vi "FisherPaykel Check SubCycle.vi"(7 "Agitate Parameters Settle Stroke":T1={"Agitate Running Time (sec)"=15, "Direction (CW or CCW)"="1", "RampUpTime (1-600ms)"=250, "TargetSpeed (0-200RPM)"=726, "PlateauTime (0-1800ms 10ms Increment)"=1000, "PauseTime (0-1800ms 10ms Increment)"=600} {"PauseTime (0-1800ms 10ms Increment)" step=10; "PlateauTime (0-1800ms 10ms Increment)" step=10; "TargetSpeed (0-200RPM)" max=1600 step=1; "RampUpTime (1-600ms)" max=600 step=10; "Agitate Running Time (sec)" step=1}, 8 "Error In":errorcluster, 9 "Agitate Parameters":T1={"Agitate Running Time (sec)"=0, "Direction (CW or CCW)"="0", "RampUpTime (1-600ms)"=0, "TargetSpeed (0-200RPM)"=0, "PlateauTime (0-1800ms 10ms Increment)"=0, "PauseTime (0-1800ms 10ms Increment)"=0} {"PauseTime (0-1800ms 10ms Increment)" step=10; "PlateauTime (0-1800ms 10ms Increment)" step=10; "TargetSpeed (0-200RPM)" max=1600 step=1; "RampUpTime (1-600ms)" max=600 step=10; "Agitate Running Time (sec)" step=1}, 10 "Spin Profile":T3={"Target Speed (RPM)"=23, "Acceleration Rate - (10 Slowest/1000 Fastest)"=10, "Running Time (s)"=20, "Direction (CW or CCW)"=""} {"Running Time (s)" step=1; "Acceleration Rate - (10 Slowest/1000 Fastest)" min=10 max=1000 step=1; "Target Speed (RPM)" min=23 max=1600 step=1}, 11 "ERD Array":string[][](array[string])=[["Motor Profile Status (0xF0B7)", "Started"], ["Motor Profile (0xF0B7)", "9"], ["Motor Mode (0xF0B1)", "Idle"], ["Mode Shift Status (0xFF22)", "Agitate State"], ["Sub-Cycle (0xF07B)", "WASH"], ["Remaining Cycle Time(s) (0xF061)", "1707"], ["Target Speed (RPM) (0xF0AC)", "0"]]) -> (0 "Error Out":errorcluster, 1 "Agitate Parameters Output":T1={"Agitate Running Time (sec)"=0, "Direction (CW or CCW)"="0", "RampUpTime (1-600ms)"=0, "TargetSpeed (0-200RPM)"=0, "PlateauTime (0-1800ms 10ms Increment)"=0, "PauseTime (0-1800ms 10ms Increment)"=0} {"PauseTime (0-1800ms 10ms Increment)" step=10; "PlateauTime (0-1800ms 10ms Increment)" step=10; "TargetSpeed (0-200RPM)" max=1600 step=1; "RampUpTime (1-600ms)" max=600 step=10; "Agitate Running Time (sec)" step=1}, 2 "Spin Profile Output":T3={"Target Speed (RPM)"=23, "Acceleration Rate - (10 Slowest/1000 Fastest)"=10, "Running Time (s)"=20, "Direction (CW or CCW)"=""} {"Running Time (s)" step=1; "Acceleration Rate - (10 Slowest/1000 Fastest)" min=10 max=1000 step=1; "Target Speed (RPM)" min=23 max=1600 step=1}, 3 "States Output":string)   [LabVIEW 2016]
uses:
  Type Definitions/Fisher Paykel Motor Profile.ctl
  Type Definitions/FisherPaykel Direction CMD.ctl
  Type Definitions/Fisher Paykel Agitate Parameters.ctl
panel:
  # "Agitate Profile Parameters"
  # "Agitate Start Parameters"
  # "Agitate Profile Parameters"
  # "Agitate Start Parameters"
  # "Agitate Profile Parameters"
  # "Agitate Start Parameters"
  # "Spin Profile Parameters"
  # "Spin Start Parameters"
  # "Spin Profile Parameters"
  # "Spin Start Parameters"
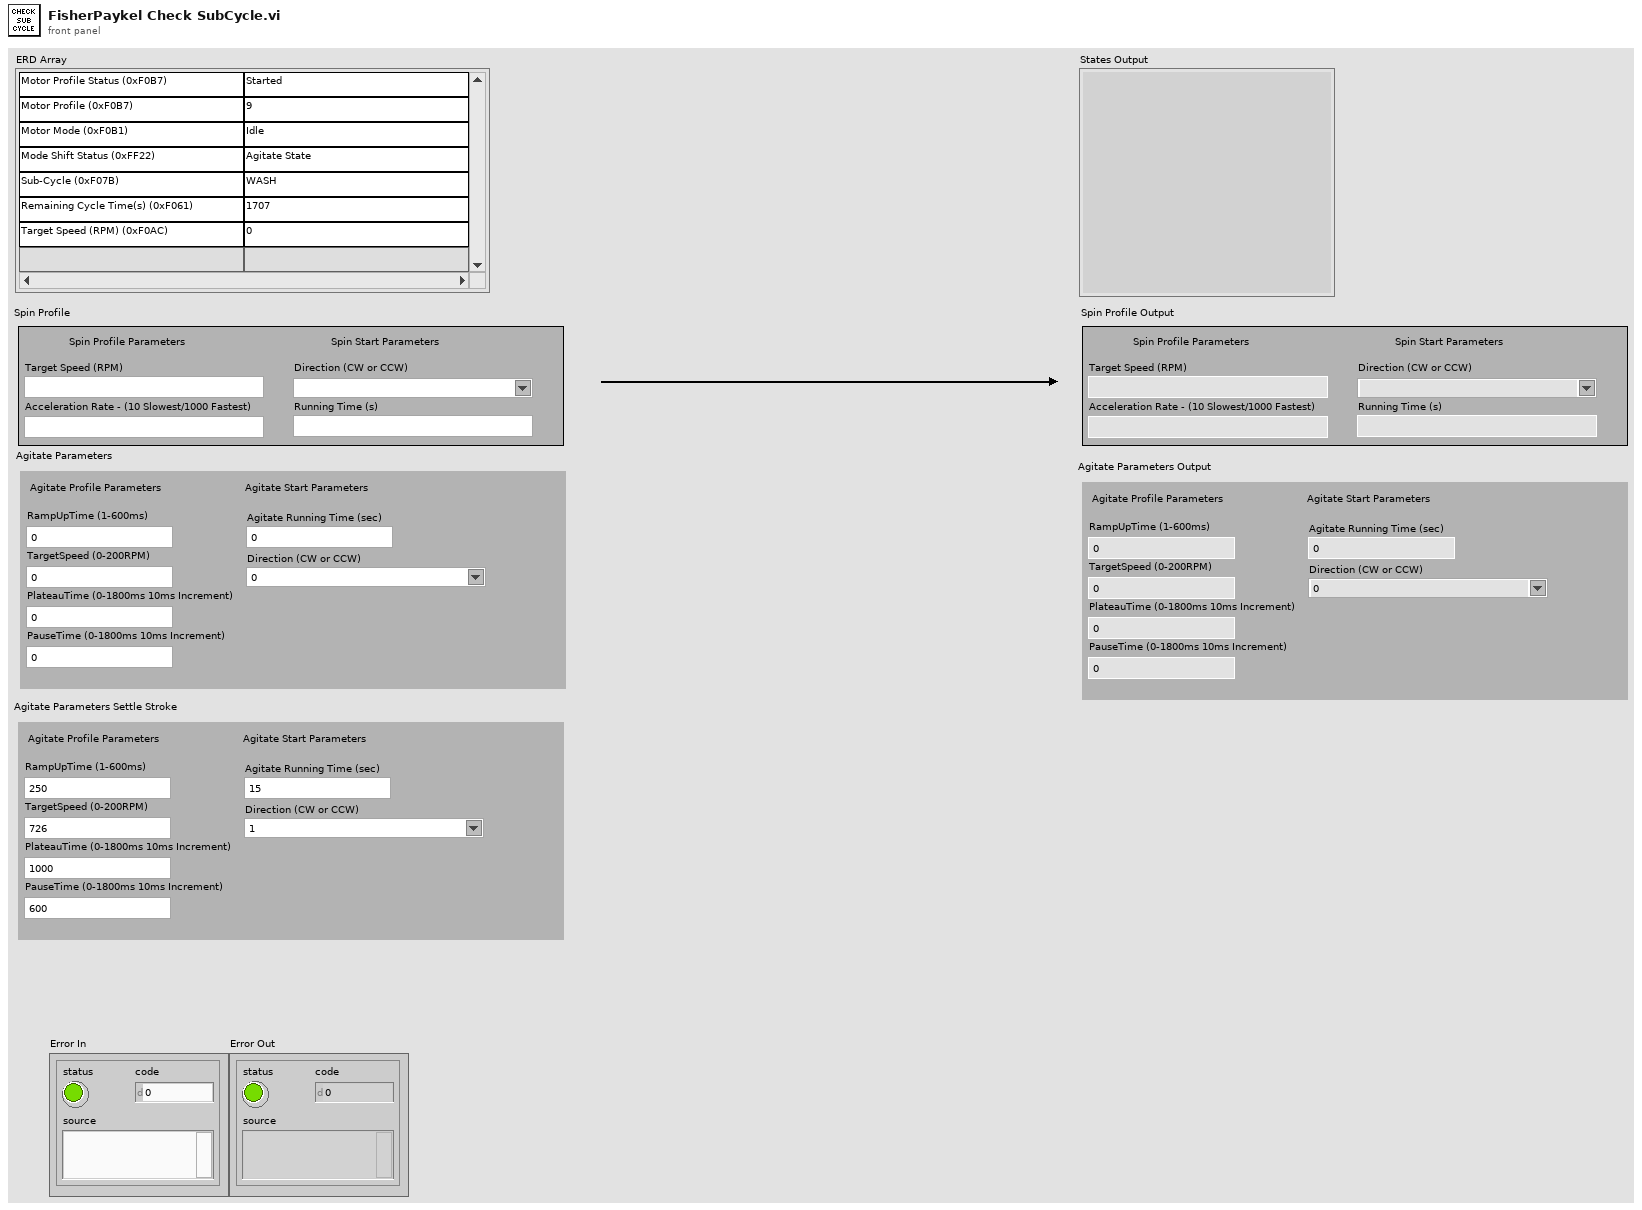
[diagram p1: front panel]
types:
  T1 = typedef "Fisher Paykel Agitate Parameters.ctl" = cluster{"Agitate Running Time (sec)":u16, "Direction (CW or CCW)":T2, "RampUpTime (1-600ms)":u16, "TargetSpeed (0-200RPM)":u16, "PlateauTime (0-1800ms 10ms Increment)":u16, "PauseTime (0-1800ms 10ms Increment)":u16}
  T2 = typedef "FisherPaykel Direction CMD.ctl" = string
  T3 = typedef "Fisher Paykel Motor Profile.ctl" = cluster{"Target Speed (RPM)":u16, "Acceleration Rate - (10 Slowest/1000 Fastest)":u16, "Running Time (s)":u16, "Direction (CW or CCW)":T2}
  T4 = typedef "FisherPaykel Motor Profile Data ERD.ctl" = cluster{"Sub-Cycle":string, "Motor Mode":string, "Mode Shift Status":string, "Target Speed (RPM)":string, "Remaining Cycle Time(s)":string, "Motor Profile Status":string, "Motor Profile Status Number":u16}
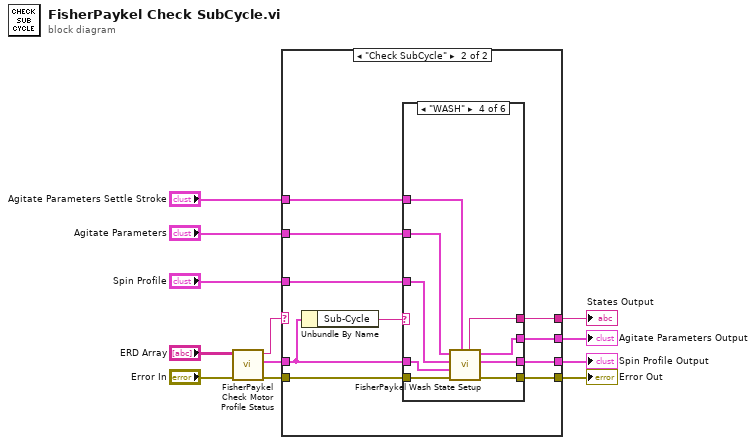
[diagram p0: block diagram]
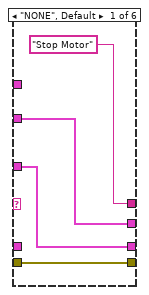
[diagram p3: hidden frame]
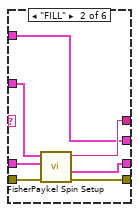
[diagram p4: hidden frame]
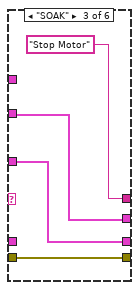
[diagram p5: hidden frame]
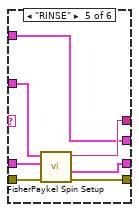
[diagram p6: hidden frame]
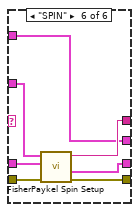
[diagram p7: hidden frame]
diagram:
  n1 = call "FisherPaykel Check Motor Profile Status.vi"("Error In"="Error In", "ERD Array"="ERD Array") -> ("Error Out"=w5:errorcluster, "Motor Profile Data"=w2:T4, "States Output"=w3:string)  [unwired: 7 in]
  n2 = case shown="\"Check SubCycle\"" w3 {
    selector: w3 -> [w16 _]
    tunnel: [w16 w26] -> w12
    tunnel: "Spin Profile" -> [w14 w25]
    tunnel: [w14 w24] -> w10
    tunnel: "Agitate Parameters" -> [w13 w23]
    tunnel: [w13 w22] -> w8
    tunnel: [w15 w21] -> w7
    tunnel: w5 -> [w15 w20]
    tunnel: w2 -> [_ w18]
    tunnel: "Agitate Parameters Settle Stroke" -> [_ w17]
    frame "Stop Motor", Default {
    }
    frame "Check SubCycle" {
      n3 = Unbundle By Name(w18) -> ("Sub-Cycle"=w19:string)
      n4 = case shown="\"WASH\"" w19 {
        tunnel: ["Stop Motor" w37 "Stop Motor" w45 w53 w62] -> w26
        tunnel: w25 -> [w27 w36 w39 w47 w57 w64]
        tunnel: [w27 w35 w39 w43 w54 w63] -> w24
        tunnel: w23 -> [w28 w32 w40 w48 w52 w59]
        tunnel: [w28 w32 w40 w44 w52 w59] -> w22
        tunnel: w20 -> [w29 w34 w38 w50 w56 w61]
        tunnel: [w29 w33 w38 w49 w55 w60] -> w21
        tunnel: w18 -> [_ w31 _ w46 w51 w58]
        tunnel: w17 -> [_ _ _ w42 _ _]
        frame "NONE", Default {
        }
        frame "FILL" {
          n5 = call "FisherPaykel Spin Setup.vi"("Error In"=w34, "Motor Profile Data"=w31, "Spin Profile in"=w36) -> ("Error Out"=w33:errorcluster, "Spin Profile out"=w35:T3, "States Out"=w37:string)  [unwired: 6 in]
        }
        frame "SOAK" {
        }
        frame "WASH" {
          n6 = call "FisherPaykel Wash State Setup.vi"("Agitate Parameters Settle Stroke"=w42, "error in (no error)"=w50, "Motor Profile Data"=w46, "Spin Profile in"=w47, "Agitate Parameters in"=w48) -> ("error out"=w49:errorcluster, "Spin Profile out"=w43:T3, "Agitate Parameters out"=w44:T1, "States Out"=w45:string)  [unwired: 3 in]
        }
        frame "RINSE" {
          n7 = call "FisherPaykel Spin Setup.vi"("Error In"=w56, "Motor Profile Data"=w51, "Spin Profile in"=w57) -> ("Error Out"=w55:errorcluster, "Spin Profile out"=w54:T3, "States Out"=w53:string)  [unwired: 6 in]
        }
        frame "SPIN" {
          n8 = call "FisherPaykel Spin Setup.vi"("Error In"=w61, "Motor Profile Data"=w58, "Spin Profile in"=w64) -> ("Error Out"=w60:errorcluster, "Spin Profile out"=w63:T3, "States Out"=w62:string)  [unwired: 6 in]
        }
      }
    }
  }
  "Error Out" <- w7
  "States Output" <- w12
  "Spin Profile Output" <- w10
  "Agitate Parameters Output" <- w8
